vi "basic - Bite Transfer.vi"() -> ()   [LabVIEW 2020]
uses:
  src/AIM664LV.lvlib
  src/_polimorphicInstances/session/Fdx Close Session (Board).vi
  src/_polimorphicInstances/session/Fdx Create Session (Generic-Board).vi
panel:
  out "Error Message":string
  out "error out":errorcluster
  in  "SrvName":string="local"
  in  "Board ID":u32
  # "ARINC 664 BITE Transfer Test"
  # "Overview: Performs some transfer tests using available port resources of one FDX board. This function will determine the number of ports on the board. If only two ports, it will test them against each other. If four ports are used, Port 1 and Port 2 will be tested against each other and Port 3 and Port 4 will be tested against each other. \nPort 1 and Port 2 must be connected with a Loop-Back cable (crossover), if available Port 3 and Port 4 must be connected with a Loop-Back cable (crossover).\nThe resources of the board under test shall be not logged in.\n\nRequirement: One AIM ARINC-664 board with installed AIM ARINC 664 BSP.\nRestrictions: None.\nInstruction:\n1. Select the Board ID (0 if you have only one board in your system).\n2. Run the VI.\n3. If no error is presented, the test was performed correctly."
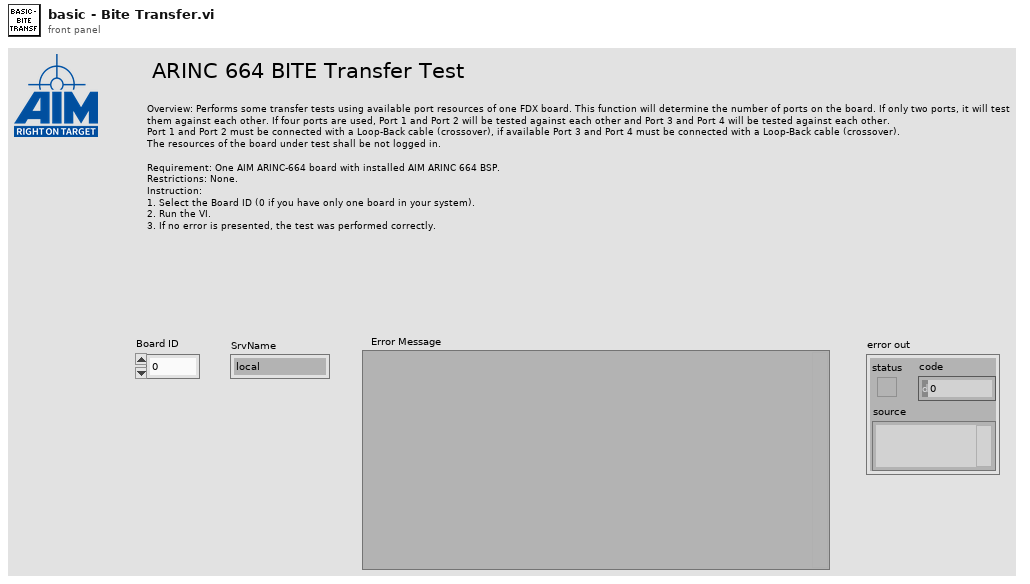
[diagram p1: front panel]
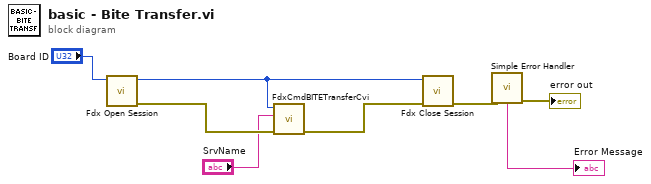
[diagram p0: block diagram]
diagram:
  n1 = call-poly "Fdx Open Session.vi"("board"="Board ID") -> ("error out"=w8:errorcluster, "InstrumentHandle_board out"=w1:u32)  [unwired: 8 in, 1 out]
  n2 = call "FdxCmdBITETransferCvi.vi"("error in"=w8, "SrvName"="SrvName", "Board_ResourceID"=w1) -> ("error out"=w7:errorcluster)  [unwired: 7 in, 1 out]
  n3 = call-poly "Fdx Close Session.vi"("error in (no error)"=w7, "InstrumentHandle_board in"=w1) -> ("error out"=w6:errorcluster)  [unwired: 9 in]
  n4 = call <vilib>:"Simple Error Handler.vi"("error in (no error)"=w6) -> ("error out"=→"error out":errorcluster, "message"=→"Error Message":string)  [unwired: 4 in, 3 out]
